vi "SineNote.vi"(1 "Duration":i32=128, 2 "Frequency":dbl=128.0) -> (0 "Waveform":dbl[](array[numeric]))   [LabVIEW 2012]
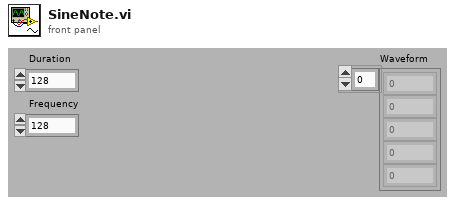
[diagram p1: front panel]
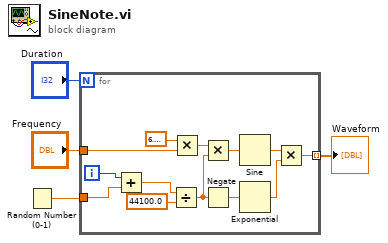
[diagram p0: block diagram]
diagram:
  n1 = Random Number (0-1)() -> (number: 0 to 1=w1:dbl)
  n2 = for {
    N: "Duration" -> [_]
    tunnel: [w15] -> w3 mode=indexing
    tunnel: "Frequency" -> [w13]
    tunnel: w1 -> [w7]
    i -> [w6]
    n3 = Add(x=w6, y=w7) -> (x+y=w5:dbl)
    n4 = Divide(x=w5, y=44100.0) -> (x/y=w9:dbl)
    n5 = Multiply(x=6.283185307179586, y=w13) -> (x*y=w10:dbl)
    n6 = Multiply(x=w10, y=w9) -> (x*y=w11:dbl)
    n7 = Negate(x=w9) -> (-x=w8:dbl)
    n8 = Sine(x=w11) -> (sin(x)=w17:dbl)
    n9 = Exponential(1:w8) -> (0:w16:dbl)
    n10 = Multiply(x=w17, y=w16) -> (x*y=w15:dbl)
  }
  "Waveform" <- w3
